vi "Membrane.vi"(0 "Насос 3":bool=TRUE, 1 "УЗ5":dbl format="%#_13g", 2 "УЗ6":dbl format="%#_13g", 3 "УЗ7":dbl format="%#_13g", 4 "Манометр":dbl format="%#_13g", 5 "Error input":bool=TRUE) -> (14 "КР2":dbl, 15 "КР3":dbl, 16 "КР5":dbl, 17 "Насос 4":bool=TRUE, 18 "КР6":dbl)   [LabVIEW 2019]
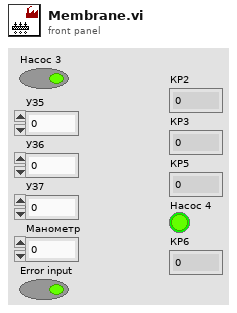
[diagram p1: front panel]
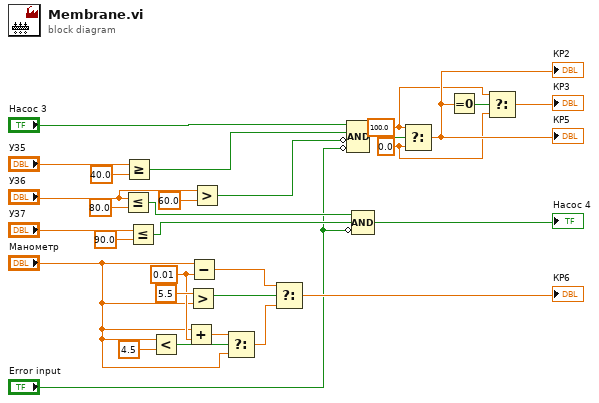
[diagram p0: block diagram]
diagram:
  w3 = 100.0 ("t")
  w2 = 0.0 ("f")
  w23 = 0.01 ("y")
  n1 = Less Or Equal?(x="УЗ6", y=80.0) -> (x <= y?=w16:bool)
  n2 = Greater Or Equal?(x="УЗ5", y=40.0) -> (x >= y?=w9:bool)
  n3 = Less Or Equal?(x="УЗ7", y=90.0) -> (x <= y?=w15:bool)
  n4 = Less?(x="Манометр", y=4.5) -> (x < y?=w22:bool)
  n5 = Add(x="Манометр", y=w23) -> (x+y=w21:dbl)
  n6 = Greater?(x=5.5, y="Манометр") -> (0:w27:bool)
  n7 = Subtract(x="Манометр", y=w23) -> (x-y=w25:dbl)
  n8 = Greater?(x="УЗ6", y=60.0) -> (0:w11:bool)
  n9 = Select(t=w21, s=w22, f="Манометр") -> (s? t:f=w19:dbl)
  n10 = Select(t=w25, s=w27, f=w19) -> (s? t:f=→"КР6":dbl)
  n11 = Compound Arithmetic op=AND("Насос 3", w9, invert w11, invert "Error input") -> (w8:bool)
  n12 = Compound Arithmetic op=AND(w16, w15, invert "Error input") -> (→"Насос 4":bool)
  n13 = Select(t=w3, s=w8, f=w2) -> (s? t:f=w5:dbl)
  "КР2" <- w5
  "КР5" <- w5
  n14 = Equal To 0?(x=w5) -> (x = 0?=w4:bool)
  n15 = Select(t=w3, s=w4, f=w2) -> (s? t:f=→"КР3":dbl)
